vi "DAQ.GetDeviceInfo.vi"(8 "error in (no error)":errorcluster, 11 "Instrument.DAQ":refnum<class "Instrument.DAQ.lvclass">) -> (0 "error out":errorcluster, 3 "Instrument.DAQ":refnum<class "Instrument.DAQ.lvclass">)   [LabVIEW 2019, in "Instrument.Lockin.lvlib" / "Instrument.DAQ.lvclass"]
uses:
  Instrument.DAQ.lvclass
  DAQmx/DAQmx.lvclass
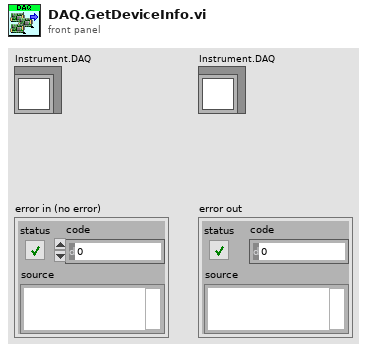
[diagram p1: front panel]
types:
  T1 = typedef "DAQmx.lvclass/DeviceInfo--Cluster.ctl" = cluster{"DeviceName":string, "DevIsSimulated":bool, "DeviceSerialNumber":u32, "ProductType":string, "ProductCategory":i32, "ProductNumber":u32, "ChassisNumber":u32, "SlotNumber":u32, "ChassisName":string, "ChassisSerialNumber":u32}
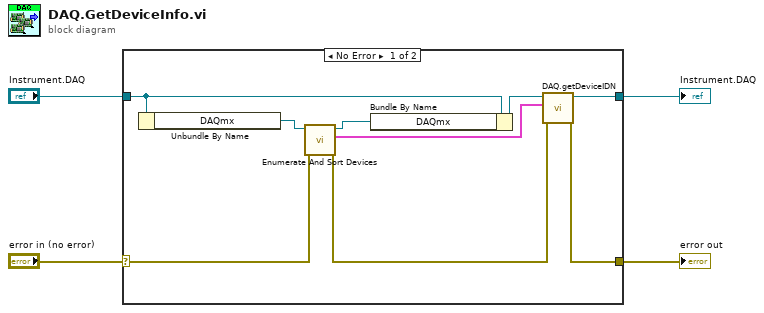
[diagram p0: block diagram]
diagram:
  n1 = case shown="No Error" "error in (no error)" {
    selector: "error in (no error)" -> [w13 w14]
    tunnel: "Instrument.DAQ" -> [w5 w15]
    tunnel: [w12 w15] -> w2
    tunnel: [w10 w14] -> w1
    frame No Error {
      n2 = Unbundle By Name(w5) -> ("DAQmx"=w8:refnum<class "DAQmx.lvclass">)
      n3 = call "Enumerate And Sort Devices.vi"("error in (no error)"=w13, "DAQmx in"=w8) -> ("error out"=w11:errorcluster, "Devices (sorted)"=w6:T1[], "DAQmx out"=w9:refnum<class "DAQmx.lvclass">)  [unwired: 7 in]
      n4 = Bundle By Name(cluster=w5, "DAQmx"=w9) -> (w7:refnum<class "Instrument.DAQ.lvclass">)
      n5 = call "DAQ.getDeviceIDN.vi"("error in (no error)"=w11, "Devices"=w6, "Instrument.DAQ"=w7) -> ("error out"=w10:errorcluster, "Instrument.DAQ out"=w12:refnum<class "Instrument.DAQ.lvclass">)  [unwired: 7 in]
    }
    frame Error {
    }
  }
  "Instrument.DAQ" <- w2
  "error out" <- w1
